vi "Handle setAllData.vi"(8 "error in (no error)":errorcluster, 10 "AllData":variant, 11 "Inst.Xeryon-Rotator in":refnum<class "Inst.Xeryon-Rotator.lvclass">) -> (0 "error out":errorcluster, 3 "Inst.Xeryon-Rotator out":refnum<class "Inst.Xeryon-Rotator.lvclass">)   [LabVIEW 2019, in "Inst.Xeryon-Rotator.lvclass"]
doc: "Override to handle \"getAll\" or \"getAllData\" commands for <b>your</b> Instrument"
uses:
  Inst.Xeryon-Rotator.lvclass
  Typedefs/Inst.Xeryon-Rotator.getAll--Cluster.ctl
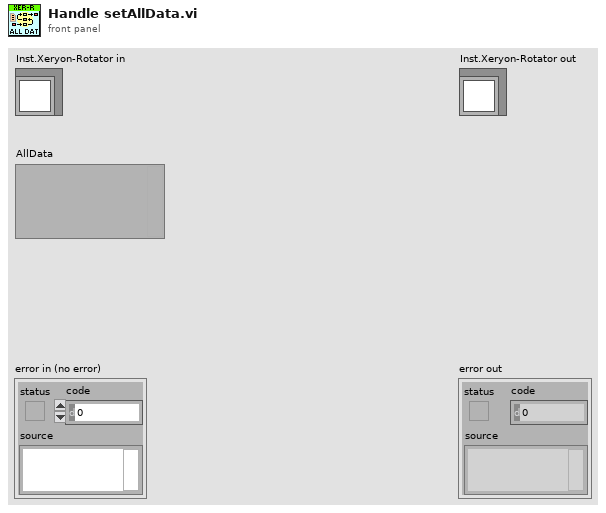
[diagram p1: front panel]
types:
  T1 = typedef "Inst.Xeryon-Rotator.lvclass/Inst.Xeryon-Rotator.getAll--Cluster.ctl" = cluster{"Encoder position [selected units]":dbl, "Desired Position [selected units]":dbl, "Status":string, "SRNO":dbl, "SOFT":dbl, "STAT":dbl, "FREQ":dbl, "OFRQ":dbl, "CURR":dbl, "SYNC":dbl, "Encoder Position [enc. units]":dbl, "Desired Position [enc. units]":dbl, "TIME":dbl, "Index Found":bool, "Left Limit":bool, "Right Limit":bool, "Position Reached":bool}
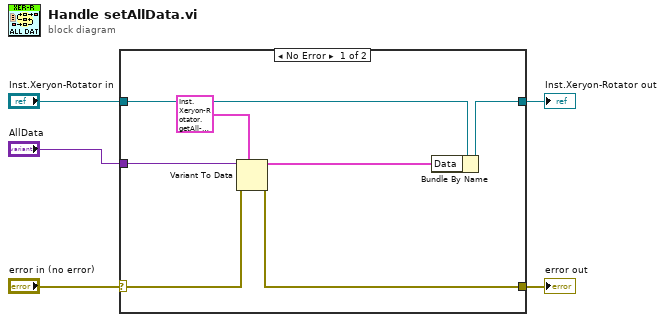
[diagram p0: block diagram]
diagram:
  n1 = case shown="No Error" "error in (no error)" {
    selector: "error in (no error)" -> [w8 w13]
    tunnel: "Inst.Xeryon-Rotator in" -> [w10 w14]
    tunnel: [w9 w14] -> w3
    tunnel: [w7 w13] -> w2
    tunnel: "AllData" -> [w6 _]
    frame No Error {
      n2 = Variant To Data(error in=w8, type=T1 {"Encoder position [selected units]"=0.0, "Desired Position [selected units]"=0.0, "Status"="", "SRNO"=0.0, "SOFT"=0.0, "STAT"=0.0, "FREQ"=0.0, "OFRQ"=0.0, "CURR"=0.0, "SYNC"=0.0, "Encoder Position [enc. units]"=0.0, "Desired Position [enc. units]"=0.0, "TIME"=0.0, "Index Found"=FALSE, "Left Limit"=FALSE, "Right Limit"=FALSE, "Position Reached"=FALSE} ("Data"), Variant=w6) -> (data=w11:T1, error out=w7:errorcluster)
      n3 = Bundle By Name(cluster=w10, "Data"=w11) -> (w9:refnum<class "Inst.Xeryon-Rotator.lvclass">)
    }
    frame Error {
    }
  }
  "error out" <- w2
  "Inst.Xeryon-Rotator out" <- w3
